vi "McP Write&Read v0.41.vi"(5 "error in (no error)":errorcluster, 6 "Timeout Limit":dbl=3.0 format="%.2f", 8 "Write String":string="X\r") -> (0 "error out":errorcluster, 1 "Timeout":bool, 2 "Error Out":bool, 3 "Read String\nshows:":string="XK= 3 I= 25078 V= 49152 \r\r\n", 4 "PortNumber":i32=1 min=0 max=5)   [LabVIEW 2020]
doc: "Send commands to the McPherson 789A-3 controller and receive returned infomation.\n\nMcPherson 789A-3 controller Needs \"\\s\\r\" to initially respond! Then terminate commands with \"\\r\"\n\nThe Serial port number is a global variable."
uses:
  Globals and TypeDefs/Global Varibal Control.vi
panel:
  out "Read String":string="XK= 3 I= 25078 V= 49152 \r\r\n"
  # "Controller Needs \"\\s\\r\" to initially respond!  Then terminate commands with \"\\r\""
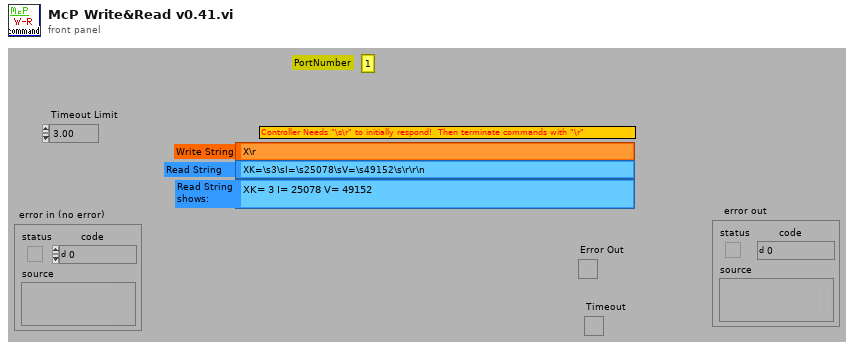
[diagram p1: front panel]
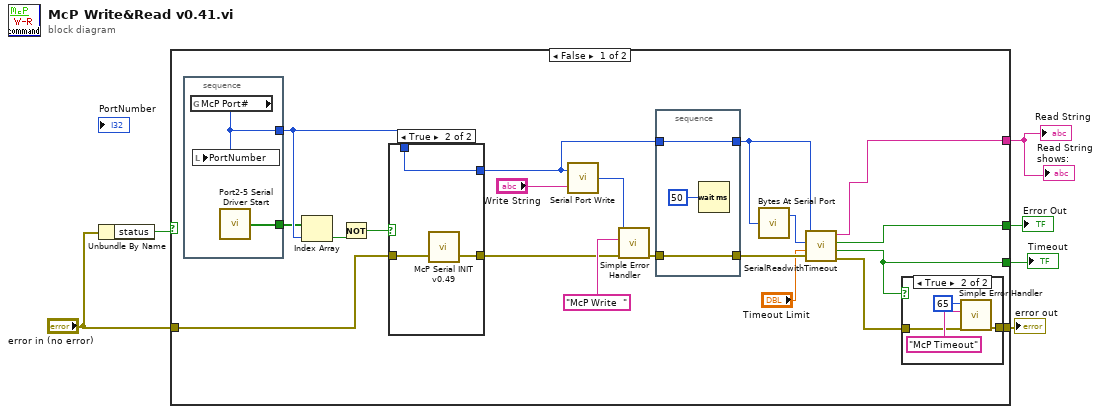
[diagram p0: block diagram]
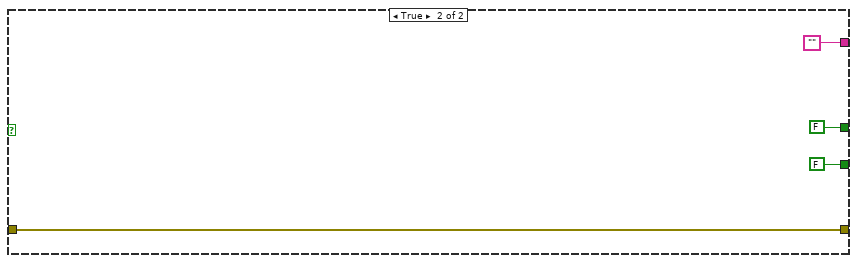
[diagram p4: hidden frame]
diagram:
  n1 = Unbundle By Name("error in (no error)") -> ("status"=w4:bool)
  n2 = case shown="False" w4 {
    tunnel: "error in (no error)" -> [w21 w45]
    tunnel: [w14 w45] -> w6
    tunnel: [w13 ""] -> w3
    tunnel: [w12 FALSE ("Error Out")] -> w2
    tunnel: [w11 FALSE ("Timeout")] -> w1
    frame False {
      n3 = stacked-sequence {
        tunnel: [w32] -> w20
        tunnel: [w33] -> w17
        frame #0 {
          n4 = global read "Global Varibal Control.vi" "McP Port#"() -> (w32:i32)
          n5 = local write "PortNumber"(w32) -> ()
          n6 = call "Port2-5 Serial Driver Start.vi"() -> ("driver opened"=w33:bool[])  [unwired: 1 in]
        }
      }
      n7 = Index Array(array=w17, index=w20) -> (element=w19:bool)
      n8 = Not(x=w19) -> (.not. x?=w10:bool)
      n9 = case shown="True" w10 {
        tunnel: w20 -> [w38 w39]
        tunnel: [w38 w39] -> w7
        tunnel: [w37 w40] -> w23
        tunnel: w21 -> [w37 w41]
        frame False {
        }
        frame True {
          n10 = call "McP Serial INIT v0.49.vi"("error in (no error)"=w41) -> ("Error out"=w40:errorcluster)  [unwired: 1 in, 1 out]
        }
      }
      n11 = call <vilib>:"Serial Port Write.vi"("string to write"="Write String", "port number"=w7) -> ("error code"=w25:i32)
      n12 = call <vilib>:"Simple Error Handler.vi"("error code (no error:0)"=w25, "error source (\" \")"="McP Write  ", "error in (no error)"=w23) -> ("error out"=w22:errorcluster)  [unwired: 2 in, 4 out]
      n13 = stacked-sequence {
        tunnel: [w35] -> w9
        tunnel: w7 -> [w35]
        tunnel: [w34] -> w18
        tunnel: w22 -> [w34]
        frame #0 {
          n14 = Wait (ms)(milliseconds to wait=u32 50) -> ()  [unwired: 1 out]
        }
      }
      n15 = call <vilib>:"Bytes At Serial Port.vi"("port number"=w9) -> ("byte count"=w8:u32)  [unwired: 1 out]
      n16 = call "SerialReadwithTimeout.vi"("error in (no error)"=w18, "Timeout Limit"="Timeout Limit", "Bytes to Read"=w8, "Port Number"=w9) -> ("error out"=w15:errorcluster, "Timeout"=w11:bool, "Error Out"=w12:bool, "Serial Read"=w13:string)
      n17 = case shown="True" w11 {
        tunnel: w15 -> [w27 w29]
        tunnel: [w27 w28] -> w14
        frame False {
        }
        frame True {
          n18 = call <vilib>:"Simple Error Handler.vi"("error code (no error:0)"=65, "error source (\" \")"="McP Timeout", "error in (no error)"=w29) -> ("error out"=w28:errorcluster)  [unwired: 2 in, 4 out]
        }
      }
    }
    frame True {
    }
  }
  "error out" <- w6
  "Read String\nshows:" <- w3
  "Read String" <- w3
  "Timeout" <- w1
  "Error Out" <- w2
